vi "Blink.vi"() -> ()   [LabVIEW 2016]
panel:
  out "Led 1":bool
  out "Led 2":bool
  in  "stop":bool
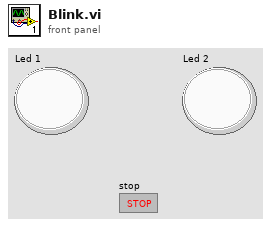
[diagram p1: front panel]
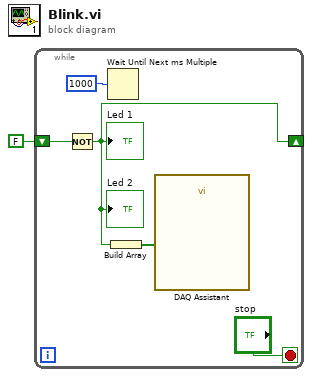
[diagram p0: block diagram]
diagram:
  n1 = while {
    shift-right: [w2] -> _
    shift-left: FALSE -> [w4]
    stop <- "stop" stop-if-true
    n2 = Not(x=w4) -> (.not. x?=w2:bool)
    "Led 2" <- w2
    "Led 1" <- w2
    n3 = Wait Until Next ms Multiple(millisecond multiple=u32 1000) -> ()  [unwired: 1 out]
    n4 = Build Array(w2) -> (w3:bool[])
    n5 = call "DAQ Assistant"("data"=w3) -> ()  [unwired: 17 in, 2 out]
  }
